vi "Read Rate A (GPM).vi"(8 "error out":errorcluster, 9 "Simulate":bool, 10 "Averages":i32=100, 11 "VISA resource name out":refnum<visa-resource-name>) -> (0 "error IO":errorcluster, 2 "GPM":dbl, 3 "VISA resource  out":refnum<visa-resource-name>)   [LabVIEW 2012, in "FEM-03.lvlib"]
uses:
  FEM-03.lvlib
  Private/Controls/Variable List.ctl
  <vilib>/Analysis/baseanly.llb/Mean (DBL).vi
  <vilib>/Analysis/NI_AALBase.lvlib
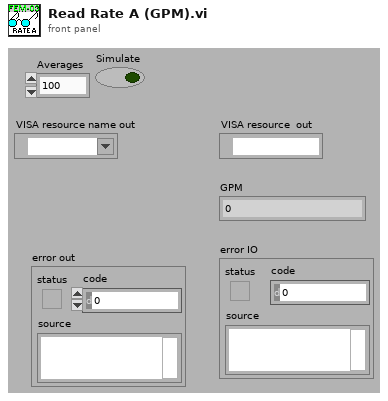
[diagram p1: front panel]
types:
  T1 = typedef "FEM-03.lvlib/Variable List.ctl" = enum16{"Rate A (PL)", "Rate A (GT)", "Job Total A", "Grand Total A", "A-KFR for Rate", "A-KFR decimal point location", "A-KFT for Total", "A-KFT decimal point location ", "A-Rate Engineering Units", "A-Total Engineering units", "A-Flow Direction", "Rate B (PL)", "Rate B (GT)", "Job Total B", "Grand Total B", "B-KFR for Rate", "B-KFR deciminal point location", "B-Rate Engineering units", "B-KFT for Total", "B-KFT decimal point location", "B-Total Engineering units", "Limit 1 Mode", "Limit1", "Margin 1 for rate limit", "Limit 2 Mode", "Limit2", "Margin 2 for rate limit", "Milli-amps Offset", "Milli-amps Out", "Analog Out Mode", "Serial Speed", "Unit Number", "Serial RESET TOTAL", "Update EEPROM", "Relay Override", "FORCE mA Output"}
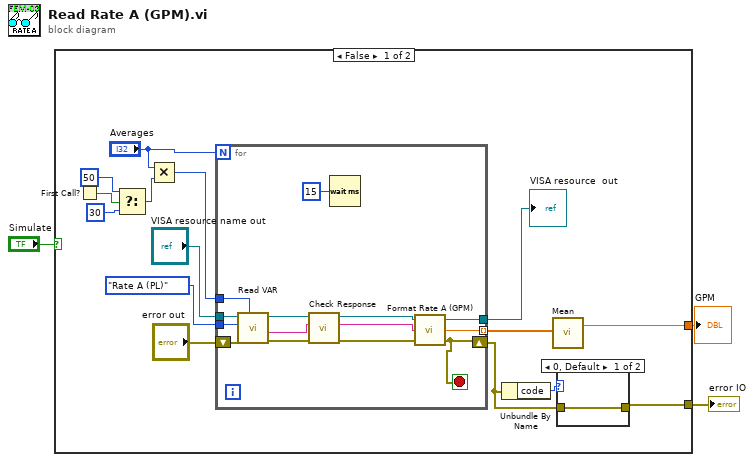
[diagram p0: block diagram]
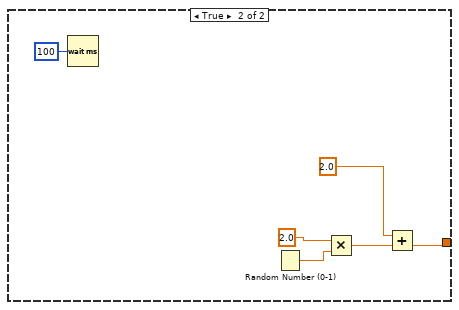
[diagram p3: hidden frame]
diagram:
  n1 = case shown="False" "Simulate" {
    tunnel: [w13 w36] -> w3
    tunnel: [w10 _] -> w1
    frame False {
      n2 = First Call?() -> (First Call?: T/F=w7:bool)
      n3 = Select(t=50 ("y"), s=w7, f=30 ("y")) -> (s? t:f=w5:i32)
      n4 = Multiply(x="Averages", y=w5) -> (x*y=w8:i32)
      n5 = for {
        N: "Averages" -> [_]
        tunnel: [w33] -> w14 mode=indexing
        tunnel: [w32] -> w18
        tunnel: Variable_List."Rate A (PL)" ("Variable to Read") -> [w25]
        tunnel: w8 -> [w24]
        tunnel: "VISA resource name out" -> [w23]
        shift-right: [w21] -> w11
        shift-left: "error out" -> [w22]
        stop <- w21 stop-if-true
        n6 = call "Read VAR.vi"("Timeout (ms)"=w24, "error in"=w22, "Variable to Read"=w25, "VISA resource name"=w23) -> ("error out"=w28:errorcluster, "Read Buffer"=w26:string, "VISA resource name out"=w27:refnum<visa-resource-name>)  [unwired: 5 in]
        n7 = call "Check Response.vi"("Error In"=w28, "Read Buffer"=w26, "VISA resource"=w27) -> ("error out"=w30:errorcluster, "Filtered Response"=w29:string, "VISA resource  out"=w31:refnum<visa-resource-name>)  [unwired: 6 in]
        n8 = Wait (ms)(milliseconds to wait=u32 15) -> ()  [unwired: 1 out]
        n9 = call "Format Rate A (GPM).vi"("error out"=w30, "Filtered Response"=w29, "VISA resource  in"=w31) -> ("error IO"=w21:errorcluster, "GPM"=w33:dbl, "VISA resource  out"=w32:refnum<visa-resource-name>)
      }
      "VISA resource  out" <- w18
      n10 = Unbundle By Name(w11) -> ("code"=w12:i32)
      n11 = call-poly <vilib>:"Mean.vi"("X"=w14) -> ("mean"=w13:dbl)  [unwired: 1 out]
      n12 = case shown="0, Default" w12 {
        tunnel: w11 -> [w19 _]
        tunnel: [w19 _] -> w10
        frame 0, Default {
        }
        frame 1073676294 {
        }
      }
    }
    frame True {
      n13 = Wait (ms)(milliseconds to wait=u32 100) -> ()  [unwired: 1 out]
      n14 = Random Number (0-1)() -> (number: 0 to 1=w39:dbl)
      n15 = Multiply(x=2.0, y=w39) -> (x*y=w38:dbl)
      n16 = Add(x=2.0, y=w38) -> (x+y=w36:dbl)
    }
  }
  "GPM" <- w3
  "error IO" <- w1
